vi "xijk_create_example_list.vi"(8 "error in":errorcluster, 11 "path":path) -> (0 "error out":errorcluster, 1 "example list array out":string[](array[string]), 3 "filepath array out":path[](array[path]))   [LabVIEW 2010]
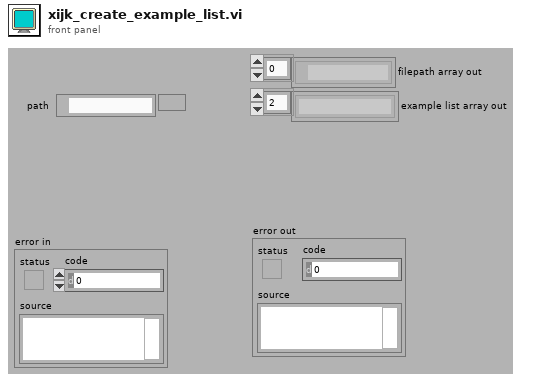
[diagram p1: front panel]
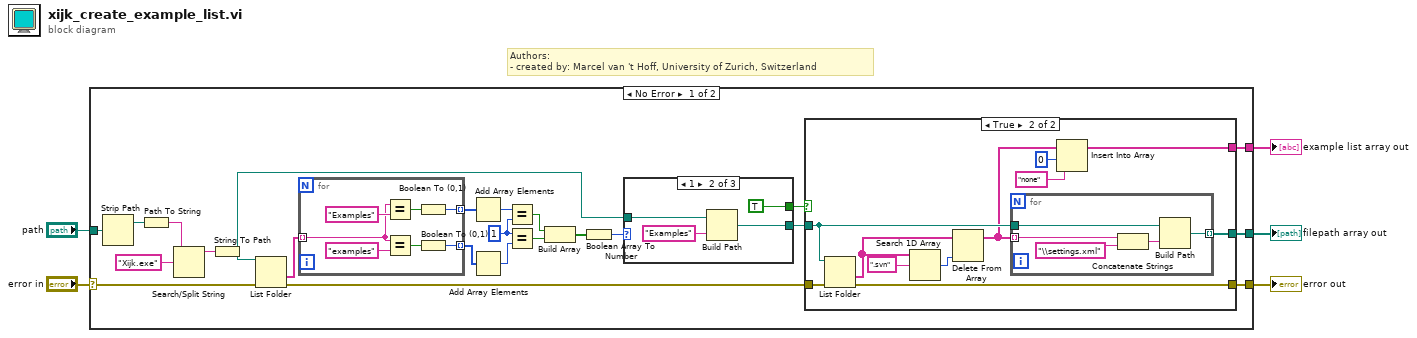
[diagram p0: block diagram]
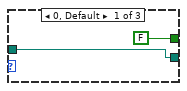
[diagram p3: hidden frame]
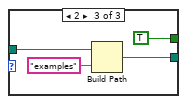
[diagram p4: hidden frame]
diagram:
  # "Authors: \n- created by: Marcel van 't Hoff, University of Zurich, Switzerland"
  n1 = case shown="No Error" "error in" {
    selector: "error in" -> [w9 w62]
    tunnel: [w28 _] -> w5
    tunnel: [w27 _] -> w4
    tunnel: [w10 w62] -> w3
    tunnel: "path" -> [w7 _]
    frame No Error {
      w23 = i16 1 ("y")
      n2 = Strip Path(path=w7) -> (stripped path=w12:path)  [unwired: 1 out]
      n3 = Path To String(path=w12) -> (string=w14:string)
      n4 = Search/Split String(string=w14, search string/char (-)="Xijk.exe" ("search string")) -> (substring before match=w8:string)  [unwired: 1 in, 2 out]
      n5 = String To Path(string=w8) -> (path=w6:path)
      n6 = List Folder(path=w6, error in=w9) -> (folder names=w15:string[], error out=w11:errorcluster)  [unwired: 4 out]
      n7 = for {
        tunnel: w15 -> [w49] mode=indexing
        tunnel: [w48] -> w26 mode=indexing
        tunnel: [w45] -> w24 mode=indexing
        n8 = Equal?(x=w49, y="Examples") -> (x = y?=w47:bool)
        n9 = Equal?(x=w49, y="examples") -> (x = y?=w46:bool)
        n10 = Boolean To (0,1)(Boolean=w47) -> (0, 1=w48:i16)
        n11 = Boolean To (0,1)(Boolean=w46) -> (0, 1=w45:i16)
      }
      n12 = Add Array Elements(numeric array=w26) -> (sum=w25:i16)
      n13 = Add Array Elements(numeric array=w24) -> (sum=w22:i16)
      n14 = Equal?(x=w25, y=w23) -> (x = y?=w21:bool)
      n15 = Equal?(x=w23, y=w22) -> (x = y?=w20:bool)
      n16 = Build Array(w21, w20) -> (w18:bool[])
      n17 = Boolean Array To Number(Boolean array=w18) -> (number=w19:u32)
      n18 = case shown="1" w19 {
        tunnel: w6 -> [w53 w56 w60]
        tunnel: [w53 w55 w59] -> w17
        tunnel: [FALSE TRUE TRUE] -> w16
        frame 0, Default {
        }
        frame 1 {
          n19 = Build Path(base path=w56, name or relative path="Examples" ("y")) -> (appended path=w55:path)
        }
        frame 2 {
          n20 = Build Path(base path=w60, name or relative path="examples" ("y")) -> (appended path=w59:path)
        }
      }
      n21 = case shown="True" w16 {
        tunnel: w17 -> [_ w39]
        tunnel: [_ w35] -> w27
        tunnel: [_ w30] -> w28
        tunnel: w11 -> [_ w34]
        tunnel: [_ w33] -> w10
        frame False {
        }
        frame True {
          n22 = List Folder(path=w39, error in=w34) -> (folder names=w36:string[], error out=w33:errorcluster)  [unwired: 4 out]
          n23 = Search 1D Array(1D array=w36, element=".svn") -> (index of element=w37:i32)  [unwired: 1 in]
          n24 = Delete From Array(array=w36, index=w37) -> (array with subset deleted=w29:string[])  [unwired: 1 in, 1 out]
          n25 = for {
            tunnel: w29 -> [w40] mode=indexing
            tunnel: w39 -> [w42]
            tunnel: [w41] -> w35 mode=indexing
            n26 = Concatenate Strings(w40, "\\settings.xml" ("chaîne")) -> (w43:string)
            n27 = Build Path(base path=w42, name or relative path=w43) -> (appended path=w41:path)
          }
          n28 = Insert Into Array(array=w29, index=0, new element="none" ("new element/subarray")) -> (w30:string[])
        }
      }
    }
    frame Error {
    }
  }
  "example list array out" <- w5
  "filepath array out" <- w4
  "error out" <- w3
